vi "DataFrom_ini (SubVI).vi"(0 "appended path":path, 2 "UUT":string, 5 "error in (no error)":errorcluster) -> (8 "ProductRev":string, 10 "PN":string, 11 "ParamVersion":string, 14 "UUT SoftwareVer":string, 15 "Element To Insert In ATR":string[](array[string]), 16 "Next SN":i32, 17 "FileName":string, 19 "error out":errorcluster)   [LabVIEW 2017]
uses:
  <vilib>/Utility/config.llb/Read Key (String).vi
  <vilib>/Utility/config.llb/NI_LVConfig.lvlib
panel:
  out "found?":bool
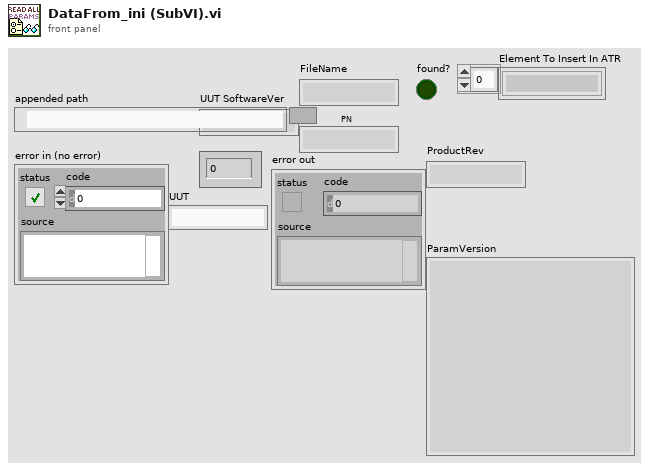
[diagram p1: front panel]
types:
  T1 = typedef "NI_LVConfig.lvlib/Config Data RefNum.ctl" = refnum<k1>
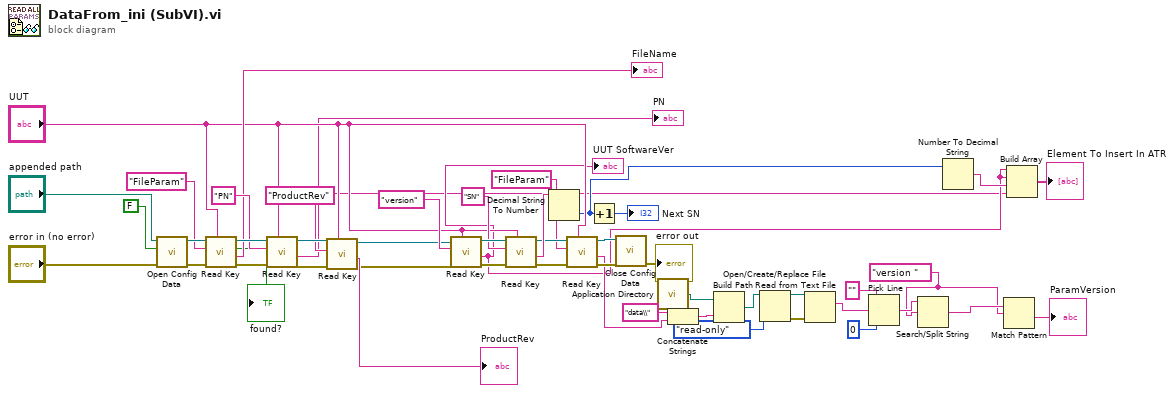
[diagram p0: block diagram]
diagram:
  w15 = "version " ("search string/char (-)")
  n1 = call <vilib>:"Open Config Data.vi"("error in (no error)"="error in (no error)", "create file if necessary (T)"=FALSE, "configuration file path"="appended path") -> ("error out"=w38:errorcluster, "refnum"=w41:T1)  [unwired: 7 out]
  n2 = call-poly <vilib>:"Read Key.vi"("section"="UUT", "error in (no error)"=w38, "key"="FileParam", "refnum"=w41) -> ("error out"=w39:errorcluster, "value"=→"FileName":string, "found?"=→"found?":bool, "refnum out"=w40:T1)  [unwired: 2 in, 2 out]
  n3 = call-poly <vilib>:"Read Key.vi"("section"="UUT", "error in (no error)"=w39, "key"="PN", "refnum"=w40) -> ("error out"=w11:errorcluster, "value"=w2:string, "refnum out"=w12:T1)  [unwired: 2 in, 3 out]
  "PN" <- w2
  n4 = call-poly <vilib>:"Read Key.vi"("section"="UUT", "error in (no error)"=w11, "key"="ProductRev", "refnum"=w12) -> ("error out"=w6:errorcluster, "value"=→"ProductRev":string, "refnum out"=w7:T1)  [unwired: 2 in, 3 out]
  n5 = call-poly <vilib>:"Read Key.vi"("section"="UUT", "error in (no error)"=w6, "key"="version", "refnum"=w7) -> ("error out"=w44:errorcluster, "value"=w3:string, "refnum out"=w45:T1)  [unwired: 2 in, 3 out]
  "UUT SoftwareVer" <- w3
  n6 = call-poly <vilib>:"Read Key.vi"("section"="UUT", "error in (no error)"=w44, "key"="SN", "refnum"=w45) -> ("error out"=w32:errorcluster, "value"=w49:string, "refnum out"=w31:T1)  [unwired: 2 in, 3 out]
  n7 = Decimal String To Number(string=w49) -> (number=w4:i32)  [unwired: 2 in, 1 out]
  n8 = call-poly <vilib>:"Read Key.vi"("section"="UUT", "error in (no error)"=w32, "key"="FileParam", "refnum"=w31) -> ("error out"=w29:errorcluster, "value"=w24:string, "refnum out"=w30:T1)  [unwired: 2 in, 3 out]
  n9 = Increment(x=w4) -> (x+1=→"Next SN":i32)
  n10 = call <vilib>:"Close Config Data.vi"("error in (no error)"=w29, "refnum"=w30) -> ("error out"=→"error out":errorcluster)  [unwired: 8 in, 1 out]
  n11 = call <vilib>:"Application Directory.vi"() -> ("Application Directory"=w27:path)
  n12 = Concatenate Strings("data\\" ("string"), w24) -> (w26:string)
  n13 = Build Path(base path=w27, name or relative path=w26) -> (appended path=w23:path)
  n14 = Open/Create/Replace File(file path (use dialog)=w23, access (0:read/write)=enum16{"read/write", "read-only", "write-only"}."read-only") -> (refnum out=w20:refnum<file>, error out=w21:errorcluster)  [unwired: 4 in, 1 out]
  n15 = Read from Text File(file (use dialog)=w20, error in=w21) -> (text=w13:string)  [unwired: 2 in, 3 out]
  n16 = Pick Line(string ("")="", multi-line string=w13, line index=0) -> (output string=w17:string)
  n17 = Search/Split String(string=w17, search string/char (-)=w15) -> (match + rest of string=w16:string)  [unwired: 1 in, 2 out]
  n18 = Number To Decimal String(number=w4) -> (decimal integer string=w5:string)  [unwired: 1 in]
  n19 = Match Pattern(string=w16, regular expression=w15) -> (after substring=→"ParamVersion":string)  [unwired: 1 in, 3 out]
  n20 = Build Array(w3, w3, w5, w2) -> (→"Element To Insert In ATR":string[])
